vi "S2C_5190CR_Proc_GetClusterValues.vi"(8 "Error In":errorcluster, 9 "ExeRef":refnum<vi>) -> (0 "Error Out":errorcluster, 3 "Settings":string[][](array[string]))   [LabVIEW 2015]
doc: "Retrieves command cluster control values and formats them for a command request transmission."
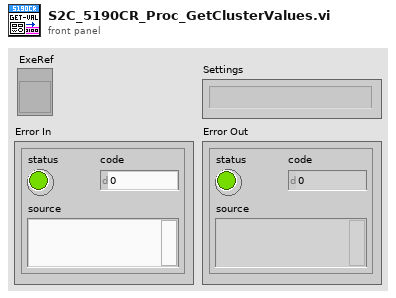
[diagram p1: front panel]
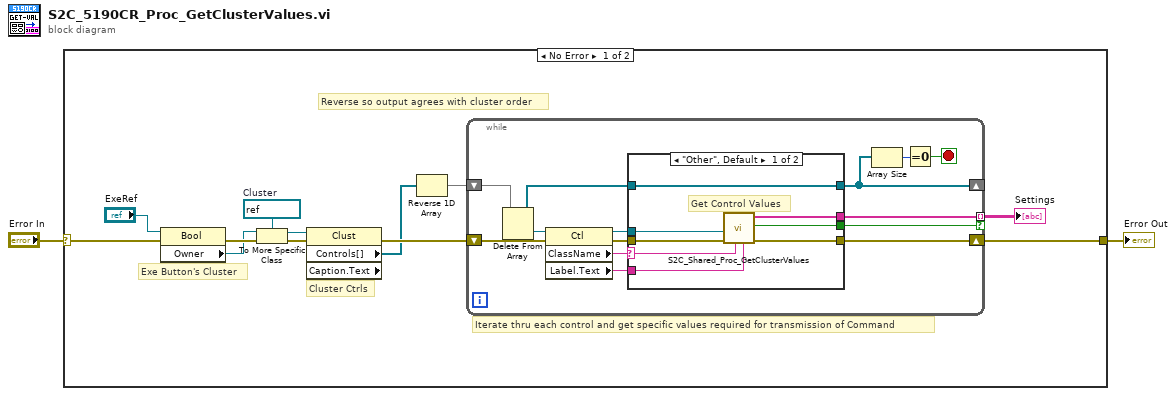
[diagram p0: block diagram]
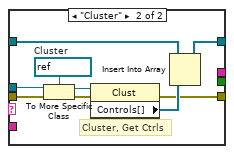
[diagram p2: hidden frame]
diagram:
  n1 = case shown="No Error" "Error In" {
    selector: "Error In" -> [w13 w46]
    tunnel: [w4 w46] -> w1
    frame No Error {
      w10 = refnum<vi> refnum  # Cluster
      # "Reverse so output agrees with cluster order"
      # "Iterate thru each control and get specific values required for transmission of Command"
      # "Cluster Ctrls"
      # "Exe Button's Cluster"
      n2 = property class="Bool"(reference="ExeRef", error in=w13) -> (error out=w12:errorcluster, "Owner"=w11:refnum<vi>)  [unwired: 1 out]
      n3 = To More Specific Class(target class=w10, reference=w11, error in=w12) -> (specific class reference=w8:refnum<vi>, error out=w9:errorcluster)
      n4 = property class="Clust" props=["Controls[]", "Caption", "Text"](reference=w8, error in=w9) -> (error out=w7:errorcluster, "Controls[]"=w6:refnum<vi>[])  [unwired: 2 out]
      n5 = Reverse 1D Array(array=w6) -> (reversed array=w5:refnum<vi>[])
      n6 = while {
        shift-right: [w22] -> _
        shift-left: w5 -> [w28]
        shift-right: [w19] -> w4
        shift-left: w7 -> [w27]
        tunnel: [w17] -> w3 mode=indexing if=w16
        stop <- w20 stop-if-true
        n7 = Delete From Array(array=w28) -> (deleted portion=w26:refnum<vi>, array with subset deleted=w23:refnum<vi>[])  [unwired: 2 in]
        n8 = property class="Ctl"(reference=w26, error in=w27) -> (reference out=w18:refnum<vi>, error out=w25:errorcluster, "ClassName"=w24:string, "Label.Text"=w15:string)
        n9 = case shown="\"Other\", Default" w24 {
          selector: w24 -> [w34 _]
          tunnel: w25 -> [w36 w41]
          tunnel: w23 -> [w32 w40]
          tunnel: [w32 w39] -> w22
          tunnel: [w33 w38] -> w19
          tunnel: w18 -> [w35 w37]
          tunnel: [w31 _] -> w17
          tunnel: [w30 _] -> w16
          tunnel: w15 -> [w29 _]
          frame "Other", Default {
            # "Get Control Values"
            n10 = call "S2C_Shared_Proc_GetClusterValues.vi"("LabelText"=w29, "ClassName"=w34, "Error In"=w36, "CtrlRef"=w35) -> ("Error Out"=w33:errorcluster, "Valid?"=w30:bool, "Settings"=w31:string[])  [unwired: 5 in]
          }
          frame "Cluster" {
            w45 = refnum<vi> refnum  # Cluster
            # "Cluster, Get Ctrls"
            n11 = To More Specific Class(target class=w45, reference=w37, error in=w41) -> (specific class reference=w43:refnum<vi>, error out=w44:errorcluster)
            n12 = property class="Clust"(reference=w43, error in=w44) -> (error out=w38:errorcluster, "Controls[]"=w42:refnum<vi>[])  [unwired: 1 out]
            n13 = Insert Into Array(array=w40, new element=w42) -> (w39:refnum<vi>[])  [unwired: 1 in]
          }
        }
        n14 = Array Size(array=w22) -> (size(s)=w21:i32)
        n15 = Equal To 0?(x=w21) -> (x = 0?=w20:bool)
      }
      "Settings" <- w3
    }
    frame Error {
    }
  }
  "Error Out" <- w1
